vi "test freqfunc -- fucking PID.vi"(6 "pars":T3={"base (Hz)"=1000.0, "period(sec)"=10.0, "amp (Hz)"=150.0, "G base (Hz)"=1000.0, "G period(sec)"=40.0, "G amp (Hz)"=150.0, "B base (V)"=1000.0, "B period(sec)"=40.0, " B amp (V)"=150.0} {"B amp (V)" format="%#_10f"; "B period(sec)" format="%#_10f"; "B base (V)" format="%#_10f"; "G amp (Hz)" format="%#_10f"; "G period(sec)" format="%#_10f"; "G base (Hz)" format="%#_10f"; "amp (Hz)" format="%#_10f"; "period(sec)" format="%#_10f"; "base (Hz)" format="%#_10f"}, 8 "lorentzian -- basic":T1={"Amplitude"=1.0, "omega(0)"=1000.0, "Gamma"=3.0, "phase"=0.0, "Q"=300.0, "Norm  Ampl"=nan, "z (inf)"=0.0+0.0i, "4corners"={"z (-pi/2)"=9.277908004825974e-07+0.0007240755403629966i, "z(inf)"=2.6527949823343002e-05+0.0007477540585896028i, "z (pi/2)"=2.8494315967368497e-06+0.0007733542176124632i, "z center"=1.8886111986097237e-06+0.0007487148789877299i, "z(0)"=-2.2750727426123552e-05+0.000749675699385857i, "radius"=2.4658065287076567e-05}} {"z (inf)" format="%#9_9f"; "Q" format="%#9_9f"; "phase" format="%#9_9f"; "Gamma" format="%#9_9f"; "omega(0)" format="%#9_9f"}, 10 "time (sec)":dbl=-1.0 format="%#_10f") -> (0 "lorentzian -- basic -- OUT":T1={"Amplitude"=1.0, "omega(0)"=1000.0, "Gamma"=3.0, "phase"=0.0, "Q"=300.0, "Norm  Ampl"=nan, "z (inf)"=0.0+0.0i, "4corners"={"z (-pi/2)"=9.277908004825974e-07+0.0007240755403629966i, "z(inf)"=2.6527949823343002e-05+0.0007477540585896028i, "z (pi/2)"=2.8494315967368497e-06+0.0007733542176124632i, "z center"=1.8886111986097237e-06+0.0007487148789877299i, "z(0)"=-2.2750727426123552e-05+0.000749675699385857i, "radius"=2.4658065287076567e-05}} {"z (inf)" format="%#9_9f"; "Q" format="%#9_9f"; "phase" format="%#9_9f"; "Gamma" format="%#9_9f"; "omega(0)" format="%#9_9f"}, 1 "freq (Hz)":dbl=-1.0 format="%#_10f")   [LabVIEW 2017]
uses:
  lorentzian.ctl
  circle corners.ctl
  shake-parameters.ctl
panel:
  # "Gamma"
  # "backgr"
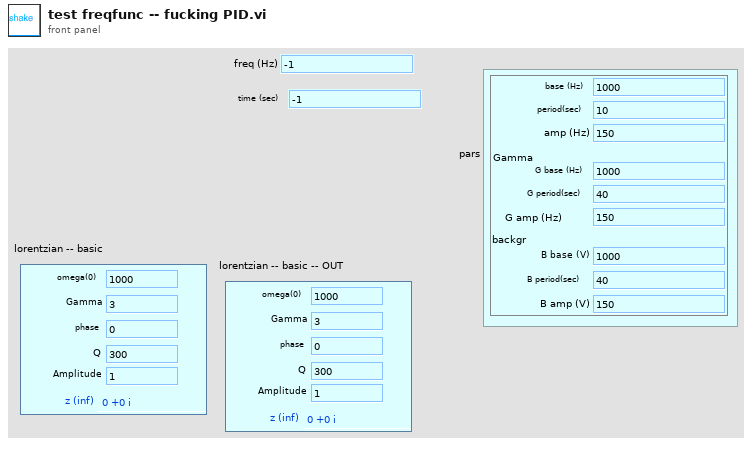
[diagram p1: front panel]
types:
  T1 = typedef "lorentzian.ctl" = cluster{"Amplitude":dbl, "omega(0)":dbl, "Gamma":dbl, "phase":dbl, "Q":dbl, "Norm  Ampl":dbl, "z (inf)":cdb, "4corners":T2}
  T2 = typedef "circle corners.ctl" = cluster{"z (-pi/2)":cdb, "z(inf)":cdb, "z (pi/2)":cdb, "z center":cdb, "z(0)":cdb, "radius":dbl}
  T3 = typedef "shake-parameters.ctl" = cluster{"base (Hz)":dbl, "period(sec)":dbl, "amp (Hz)":dbl, "G base (Hz)":dbl, "G period(sec)":dbl, "G amp (Hz)":dbl, "B base (V)":dbl, "B period(sec)":dbl, " B amp (V)":dbl}
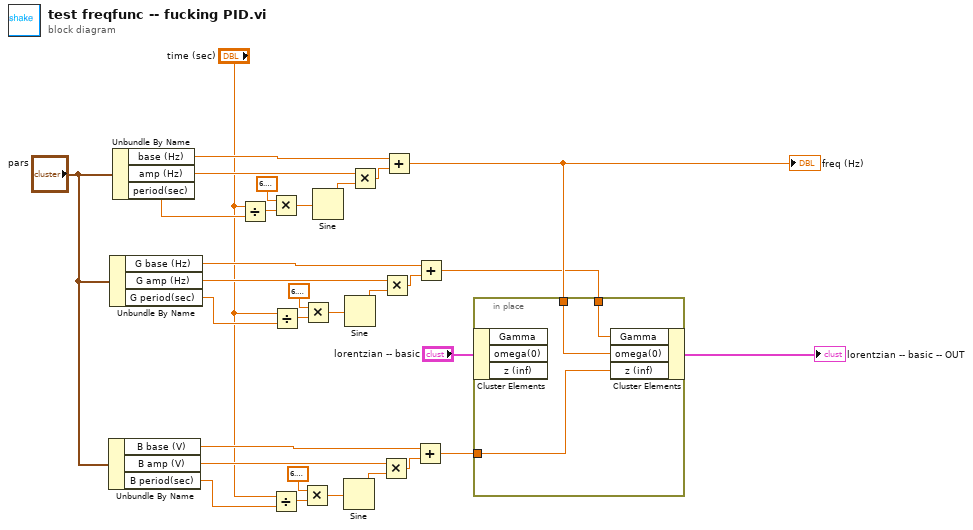
[diagram p0: block diagram]
diagram:
  n1 = Unbundle By Name("pars") -> ("B base (V)"=w6:dbl, "B amp (V)"=w5:dbl, "B period(sec)"=w4:dbl)
  n2 = Unbundle By Name("pars") -> ("G base (Hz)"=w16:dbl, "G amp (Hz)"=w15:dbl, "G period(sec)"=w14:dbl)
  n3 = Unbundle By Name("pars") -> ("base (Hz)"=w23:dbl, "amp (Hz)"=w22:dbl, "period(sec)"=w13:dbl)
  n4 = Divide(x="time (sec)", y=w13) -> (x/y=w30:dbl)
  n5 = Multiply(x=6.283185307179586, y=w30) -> (x*y=w29:dbl)
  n6 = Divide(x="time (sec)", y=w4) -> (x/y=w10:dbl)
  n7 = Divide(x="time (sec)", y=w14) -> (x/y=w20:dbl)
  n8 = Multiply(x=6.283185307179586, y=w10) -> (x*y=w9:dbl)
  n9 = Multiply(x=6.283185307179586, y=w20) -> (x*y=w19:dbl)
  n10 = Sine(x=w29) -> (sin(x)=w28:dbl)
  n11 = Sine(x=w9) -> (sin(x)=w8:dbl)
  n12 = Sine(x=w19) -> (sin(x)=w18:dbl)
  n13 = Multiply(x=w22, y=w28) -> (x*y=w27:dbl)
  n14 = Multiply(x=w5, y=w8) -> (x*y=w7:dbl)
  n15 = Multiply(x=w15, y=w18) -> (x*y=w17:dbl)
  n16 = Add(x=w23, y=w27) -> (x+y=w24:dbl)
  "freq (Hz)" <- w24
  n17 = Add(x=w6, y=w7) -> (x+y=w1:dbl)
  n18 = Add(x=w16, y=w17) -> (x+y=w12:dbl)
  n19 = in-place {
    in-place-border: w24 -> [w34]
    in-place-border: w12 -> [w33]
    in-place-border: w1 -> [w32]
    n20 = in-place-cluster #1("lorentzian -- basic") -> ()  [unwired: 3 out]
    n21 = in-place-cluster #1("Gamma"=w33, "omega(0)"=w34, "z (inf)"=w32) -> (→"lorentzian -- basic -- OUT":T1)
  }
